vi "Shooter.vi"(0 "Shooter Target RPM":dbl, 1 "Driver Shoot":bool, 2 "Shooter On":bool, 3 "Human Control":bool, 5 "Shooter RPM":dbl, 7 "Vision Turret Error":dbl, 9 "Human Turret Error":dbl, 11 "Current Hood Angle":dbl, 12 "Vision Hood Error":dbl, 13 "Human Hood Error":dbl) -> (4 "Shooter Ready":bool, 6 "Shooter Voltage":dbl, 8 "Indexer Voltage":dbl, 10 "Turret Voltage":dbl, 15 "Hood Angle":dbl)   [LabVIEW 2016]
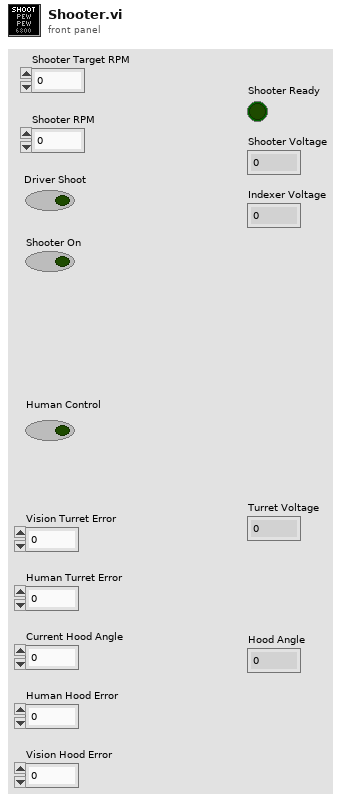
[diagram p1: front panel]
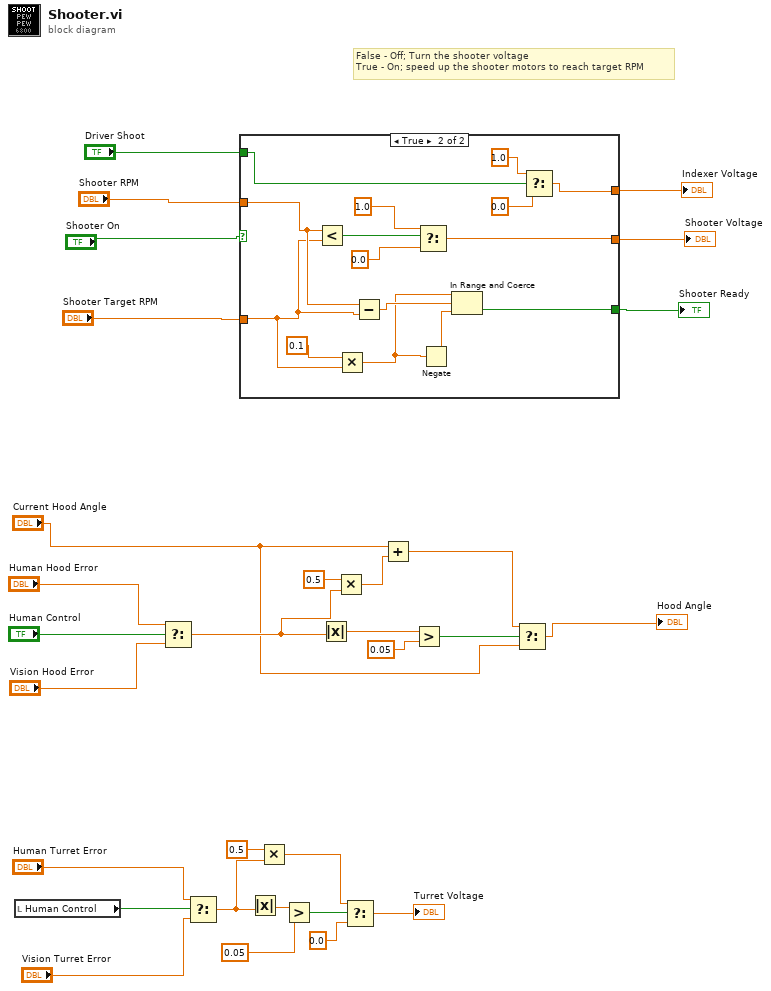
[diagram p0: block diagram]
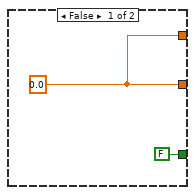
[diagram p2: hidden frame]
diagram:
  # "False - Off; Turn the shooter voltage\nTrue - On; speed up the shooter motors to reach target RPM"
  n1 = local read "Human Control"() -> (w11:bool)
  n2 = Select(t="Human Hood Error", s="Human Control", f="Vision Hood Error") -> (s? t:f=w14:dbl)
  n3 = Select(t="Human Turret Error", s=w11, f="Vision Turret Error") -> (s? t:f=w3:dbl)
  n4 = case shown="True" "Shooter On" {
    tunnel: "Driver Shoot" -> [_ w36]
    tunnel: "Shooter RPM" -> [_ w43]
    tunnel: [w32 w44] -> w27
    tunnel: "Shooter Target RPM" -> [_ w41]
    tunnel: [FALSE w37] -> w25
    tunnel: [w32 w33] -> w24
    frame False {
      w32 = 0.0 ("Shooter Voltage")
    }
    frame True {
      n5 = Less?(x=w43, y=w41) -> (x < y?=w47:bool)
      n6 = Multiply(x=0.1, y=w41) -> (x*y=w39:dbl)
      n7 = Subtract(x=w43, y=w41) -> (x-y=w42:dbl)
      n8 = Select(t=1.0, s=w47, f=0.0) -> (s? t:f=w44:dbl)
      n9 = Negate(x=w39) -> (-x=w38:dbl)
      n10 = In Range and Coerce(upper limit=w39, x=w42, lower limit=w38) -> (In Range?=w37:bool)  [unwired: 1 out]
      n11 = Select(t=1.0, s=w36, f=0.0) -> (s? t:f=w33:dbl)
    }
  }
  "Shooter Voltage" <- w27
  "Indexer Voltage" <- w24
  "Shooter Ready" <- w25
  n12 = Absolute Value(x=w3) -> (abs(x)=w10:dbl)
  n13 = Multiply(x=0.5, y=w3) -> (x*y=w2:dbl)
  n14 = Greater?(x=w10, y=0.05) -> (0:w8:bool)
  n15 = Absolute Value(x=w14) -> (abs(x)=w23:dbl)
  n16 = Multiply(x=0.5, y=w14) -> (x*y=w19:dbl)
  n17 = Select(t=w2, s=w8, f=0.0) -> (s? t:f=→"Turret Voltage":dbl)
  n18 = Add(x="Current Hood Angle", y=w19) -> (x+y=w18:dbl)
  n19 = Greater?(x=w23, y=0.05) -> (0:w21:bool)
  n20 = Select(t=w18, s=w21, f="Current Hood Angle") -> (s? t:f=→"Hood Angle":dbl)
